vi "arm-sim-main.vi"() -> ()   [LabVIEW 2020]
uses:
  RobotCode/Arm/ArmPositionPreset.ctl
  RobotCode/Arm/ArmGamePiecePreset.ctl
  <vilib>/Rock Robotics/WPI/ThirdParty/JAS_Junk/TrajLib/Enum/DCMOTOR_TYPES_ENUM.ctl
  <vilib>/Analysis/Matrix/Datatypes/RealMatrix.ctl
  <vilib>/Rock Robotics/WPI/ThirdParty/JAS_Junk/TrajLib/DCMotor_GetCIM.vi
  <vilib>/Rock Robotics/WPI/ThirdParty/JAS_Junk/TrajLib/DCMotor_GetAndymark9015.vi
  <vilib>/Rock Robotics/WPI/ThirdParty/JAS_Junk/TrajLib/DCMotor_GetAndymarkRs775_125.vi
  <vilib>/Rock Robotics/WPI/ThirdParty/JAS_Junk/TrajLib/DCMotor_GetBag.vi
  <vilib>/Rock Robotics/WPI/ThirdParty/JAS_Junk/TrajLib/DCMotor_GetBanebotsRs550.vi
  <vilib>/Rock Robotics/WPI/ThirdParty/JAS_Junk/TrajLib/DCMotor_GetBanebotsRs775.vi
  <vilib>/Rock Robotics/WPI/ThirdParty/JAS_Junk/TrajLib/DCMotor_GetFalcon500.vi
  <vilib>/Rock Robotics/WPI/ThirdParty/JAS_Junk/TrajLib/DCMotor_GetMiniCIM.vi
  <vilib>/Rock Robotics/WPI/ThirdParty/JAS_Junk/TrajLib/DCMotor_GetNEO.vi
  <vilib>/Rock Robotics/WPI/ThirdParty/JAS_Junk/TrajLib/DCMotor_GetNEO550.vi
  <vilib>/Rock Robotics/WPI/ThirdParty/JAS_Junk/TrajLib/DCMotor_GetRomiBuiltIn.vi
  <vilib>/Rock Robotics/WPI/ThirdParty/JAS_Junk/TrajLib/DCMotor_GetVex775Pro.vi
  <vilib>/Rock Robotics/WPI/ThirdParty/JAS_Junk/TrajLib/VI/DCMotor_GetAndymarkAM2235A.vi
  <vilib>/Rock Robotics/WPI/ThirdParty/JAS_Junk/TrajLib/VI/DCMotor_GetAndymarkAM3493.vi
  <vilib>/Rock Robotics/WPI/ThirdParty/JAS_Junk/TrajLib/LinearFilter_ResetToValue.vi
  <vilib>/Rock Robotics/WPI/ThirdParty/JAS_Junk/TrajLib/LinearFilter_Calculate.vi
  <vilib>/Rock Robotics/WPI/ThirdParty/JAS_Junk/TrajLib/DCMotor_New.vi
  <vilib>/Rock Robotics/WPI/ThirdParty/JAS_Junk/TrajLib/VI/Units_RotationsPerMinuteToRadiansPerSecond.vi
  <vilib>/Analysis/Matrix/Numeric/Conversions/Array To Matrix - RA.vi
  arm-sim-subvi/arm-sim-globals.vi
  <vilib>/Rock Robotics/WPI/ThirdParty/JAS_Junk/TrajLib/LinearFilter_MovingAverage.vi
  <vilib>/Rock Robotics/WPI/ThirdParty/JAS_Junk/TrajLib/LinearFilter_LowPassBW1.vi
  <vilib>/Rock Robotics/WPI/ThirdParty/JAS_Junk/TrajLib/LinearFilter_LowPassBW2.vi
  <vilib>/Rock Robotics/WPI/ThirdParty/JAS_Junk/TrajLib/LinearFilter_HighPassBW1.vi
  <vilib>/Rock Robotics/WPI/ThirdParty/JAS_Junk/TrajLib/LinearFilter_HighPassBW2.vi
  <vilib>/Rock Robotics/WPI/ThirdParty/JAS_Junk/TrajLib/Trajectory_Library.lvlib
  <vilib>/Analysis/Matrix/NI_Matrix.lvlib
panel:
  in  "Execute Preset":bool
  in  "Game Piece":T1
  in  "Position":T2=enum."Middle"
  in  "Tab Control":T3(tab)
  out "Lift Control Chart":T4(graph)
  out "Extend Control Chart":T4(graph)
  out "Battery Volts, Current Chart":cluster{"Output":dbl, "Output":dbl}(graph)
  out "Lift Err":bool
  out "RLEOnTarget":bool
  out "Extend at Low\nLimit":bool
  out "Ext Pos Inches":dbl
  out "Ext Err":bool
  out "Total Amps":dbl format="%17.2f"
  out "battery voltge":dbl format="%14.2f"
  out "ArmAngle_Deg":dbl format="%20.1f"
  # "PRESET"
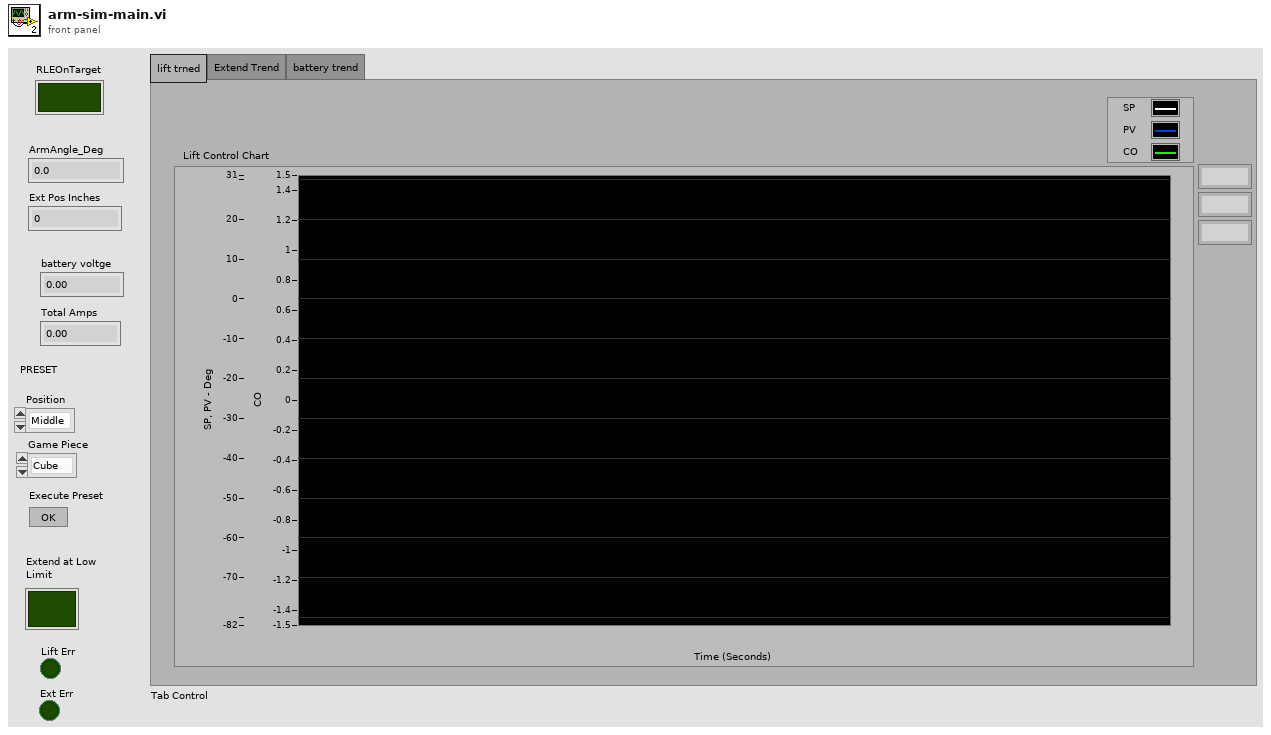
[diagram p1: front panel]
types:
  T1 = typedef "ArmGamePiecePreset.ctl" = enum16{"Cube", "Cone"}
  T2 = typedef "ArmPositionPreset.ctl" = enum16{"Upper", "Lower", "Middle", "Home", "Shelf", "Floor"}
  T3 = enum32{"lift trned", "Extend Trend", "battery trend"}
  T4 = cluster{"LiftPositionDemand(d)":dbl, "LiftPostion":dbl, "LiftMotorOutput":dbl}
  T5 = typedef "NI_Matrix.lvlib/RealMatrix.ctl" = dbl[][]
  T6 = typedef "Trajectory_Library.lvlib/DCMOTOR_TYPES_ENUM.ctl" = enum16{"CIM", "AndyMark 9015", "Andy Mark RS 775 125", "Bag", "BaneBots RS 550", "BaneBots RS 775", "Falcon 500", "Mini CIM", "NEO", "NEO 550", "Romi BuiltIn", "Vex 775 Pro", "Snow Blower AM 2235A", "Bosch Seat AM 3493"}
  T7 = typedef "Trajectory_Library.lvlib/DCMOTOR.CTL" = cluster{"nominalVoltage_Volts":dbl, "StallTorque_NM":dbl, "StallCurrent_Amps":dbl, "FreeCurrent_Amps":dbl, "FreeSpeed_RadPerSec":dbl, "R_Ohms":dbl, "KvINV_RadPerSecPerVolt":dbl, "Kt_NMPerAmp":dbl, "L_H":dbl, "Jr_KgM2":dbl}
  T8 = typedef "Trajectory_Library.lvlib/ELEVATOR_SIM.ctl" = cluster{"LinearSystemSim":T9, "GearBox":T7, "Gearing":dbl, "DrumRadius_M":dbl, "MinHeight_M":dbl, "MaxHeight_M":dbl, "CarriageMass_Kg":dbl, "SimulateGravity":bool}
  T9 = typedef "Trajectory_Library.lvlib/LINEAR_SYSTEM_SIM.ctl" = cluster{"m_Plant":T10, "m_X":T5, "m_Y":T5, "m_U":T5, "MeasureStdDev":T5}
  T10 = typedef "Trajectory_Library.lvlib/LINEAR_SYSTEM.ctl" = cluster{"m_A":T5, "m_B":T5, "m_C":T5, "m_D":T5, "States":i32, "Inputs":i32, "Outputs":i32}
  T11 = typedef "Trajectory_Library.lvlib/SINGLE_JOINT_ARM_SIM.ctl" = cluster{"Arm_LinearSystem":T9, "GearBox":T7, "Gearing":dbl, "R_ArmLength_M":dbl, "MinAngle_Rad":dbl, "MaxAngle_Rad":dbl, "SimulateGravity":bool}
  T12 = enum16{"Moving Average", "Low Pass 1st Order Butterworth", "Low Pass 2nd Order Butterworth", "High Pass 1st Order Butterworth", "High Pass 2nd Order Butterworth"}
  T13 = cluster{"ExtendPositonDemand(in)":dbl, "ExtendPostion":dbl, "ExtendMotorOutput":dbl}
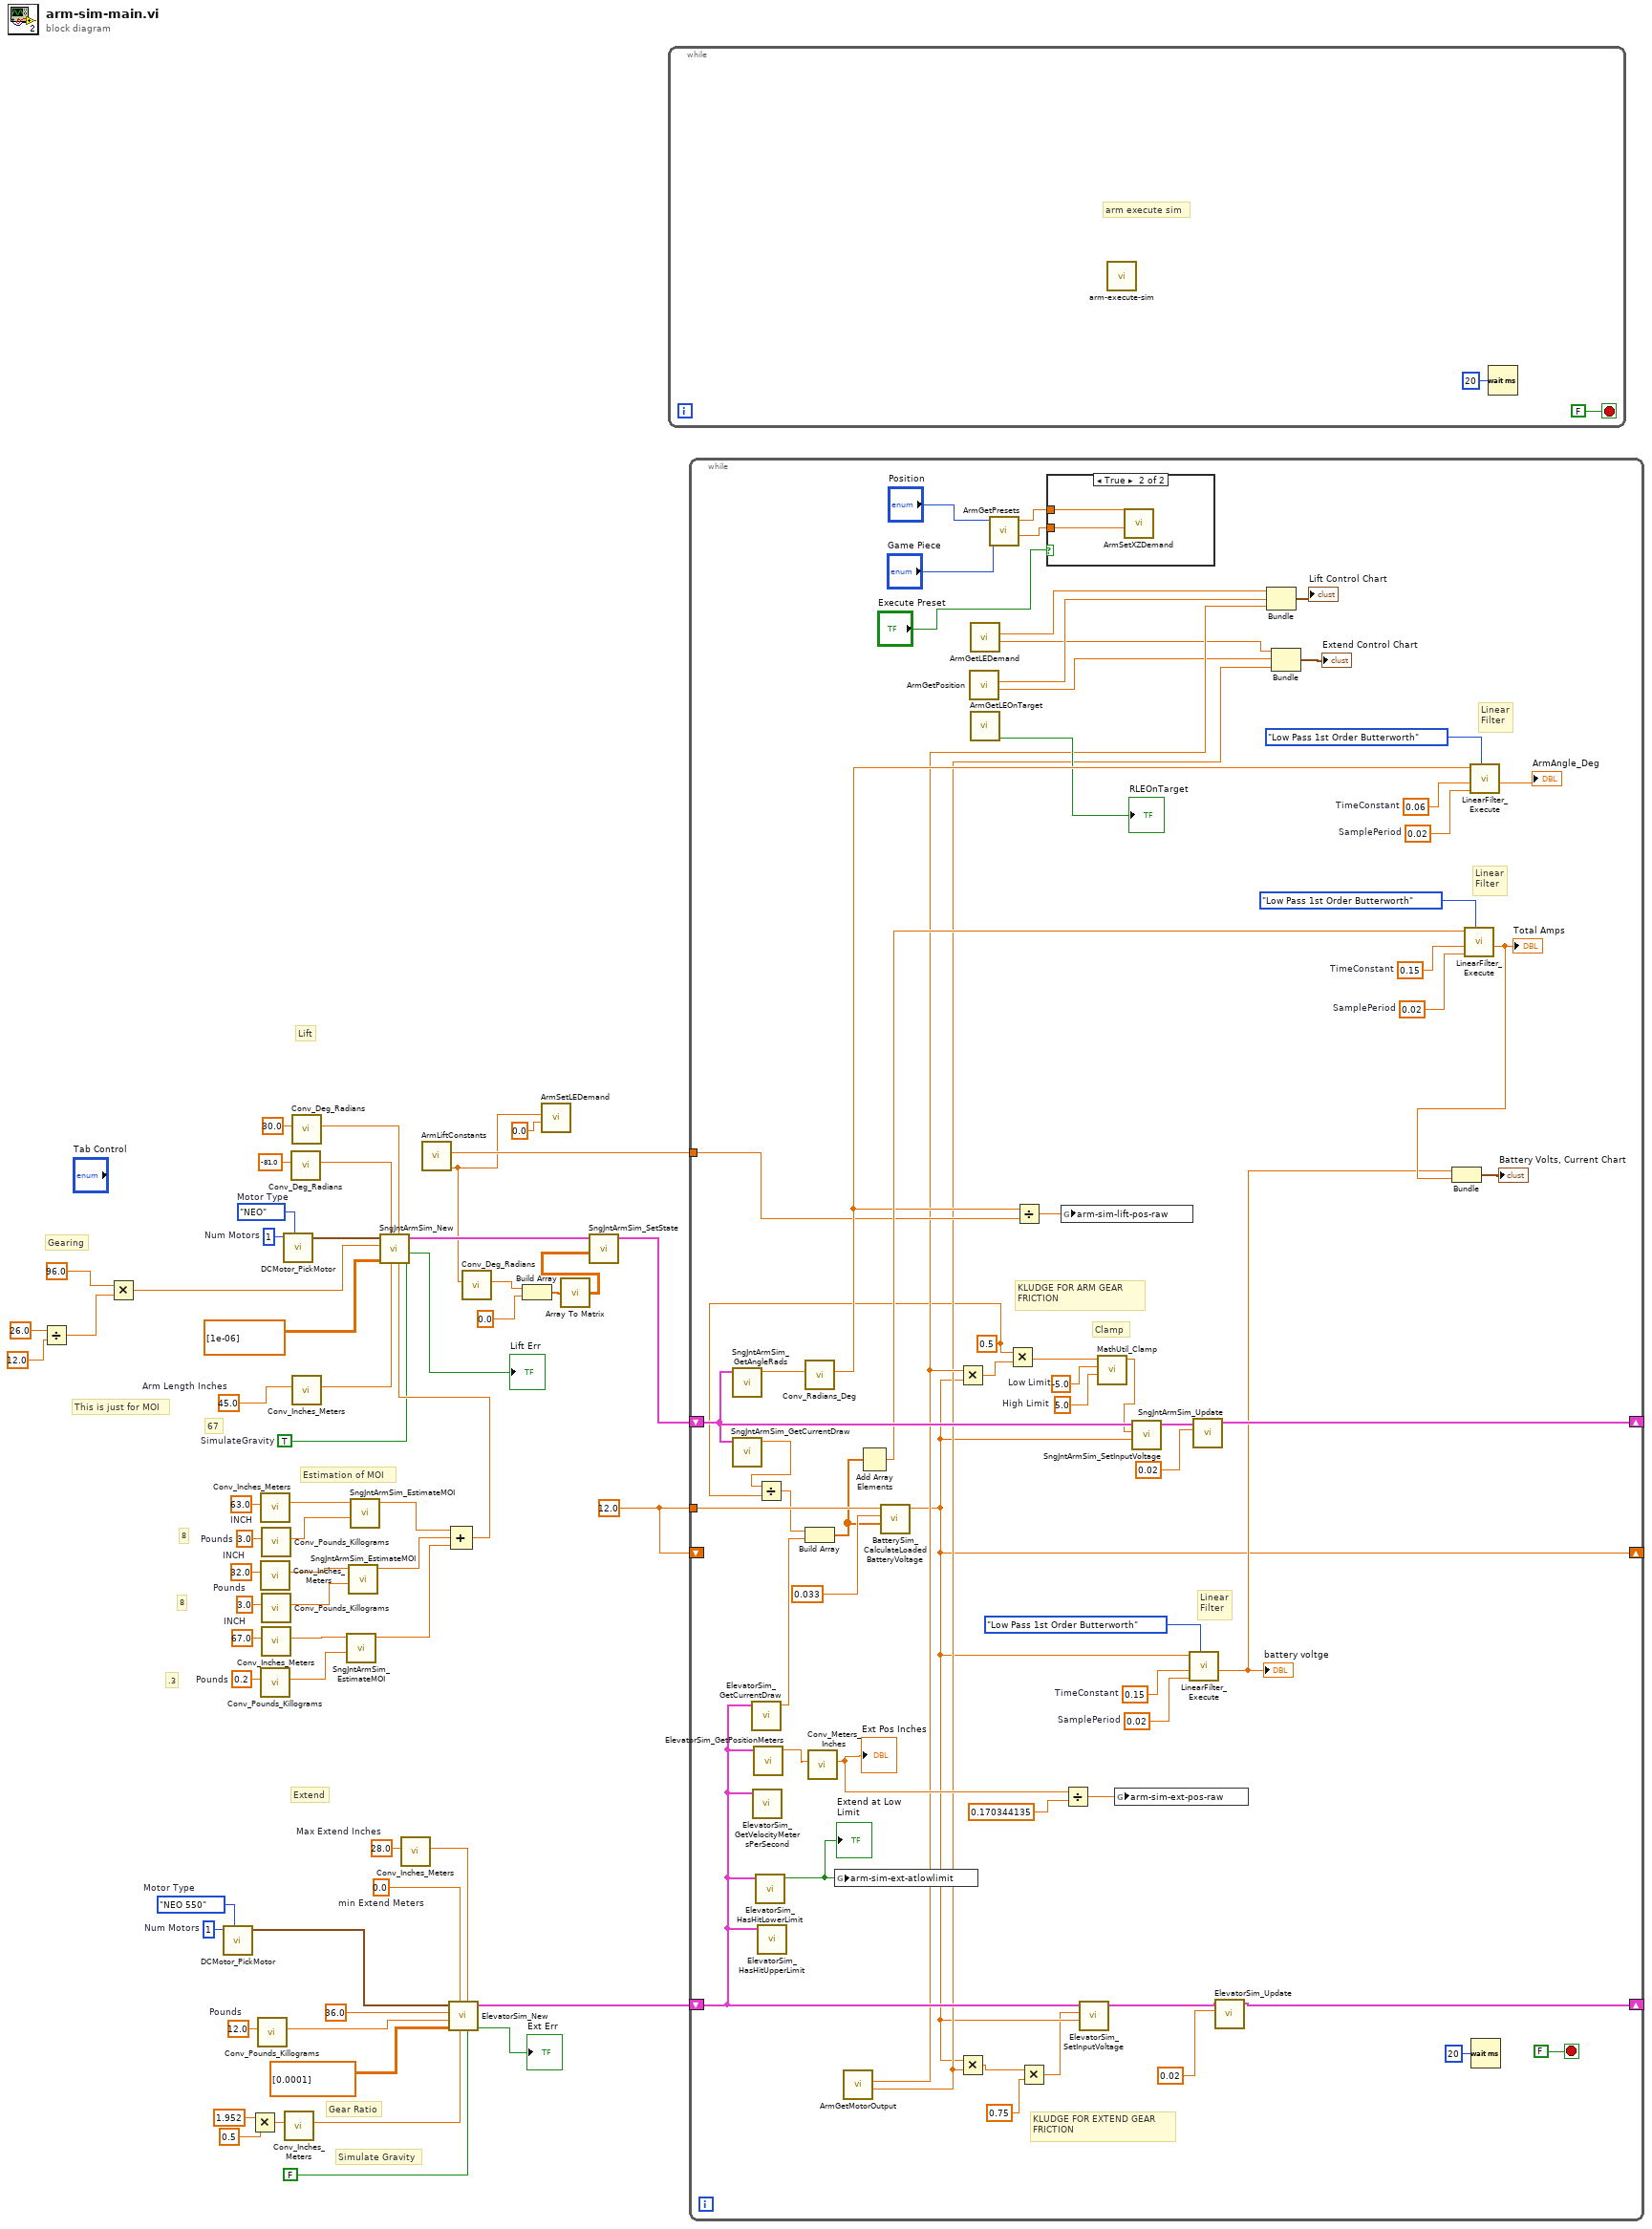
[diagram p0: block diagram]
diagram:
  w13 = 12.0  # Pounds
  w23 = 1  # Num Motors
  w22 = DCMOTOR_TYPES_ENUM."NEO 550"  # Motor Type
  w25 = 28.0  # Max Extend Inches
  w26 = 0.0  # min Extend Meters
  w35 = 12.0
  w40 = 3.0  # Pounds
  w41 = 3.0  # Pounds
  w42 = 0.2  # Pounds
  w43 = 67.0  # INCH
  w44 = 63.0  # INCH
  w45 = 32.0  # INCH
  w54 = TRUE  # SimulateGravity
  w57 = 45.0  # Arm Length Inches
  w60 = 1  # Num Motors
  w59 = DCMOTOR_TYPES_ENUM."NEO"  # Motor Type
  # "67"
  # "Simulate Gravity"
  # "Gear Ratio"
  # "Extend"
  # ".3"
  # "8"
  # "8"
  # "This is just for MOI"
  # "Estimation of MOI"
  # "Gearing"
  # "Lift"
  n1 = Divide(x=26.0, y=12.0) -> (x/y=w29:dbl)
  n2 = Multiply(x=96.0, y=w29) -> (x*y=w28:dbl)
  n3 = call <vilib>:"DCMotor_PickMotor.vi"("DCMOTOR_TYPES"=w22, "Num Motors"=w23) -> ("DCMOTOR"=w21:T7)  [unwired: 9 in]
  n4 = Multiply(x=1.952 ("INCH"), y=0.5) -> (x*y=w17:dbl)
  n5 = call <vilib>:"Conv_Pounds_Killograms.vi"("Pounds"=w13) -> ("Killograms"=w12:dbl)  [unwired: 10 in]
  n6 = call <vilib>:"Conv_Inches_Meters.vi"("INCH"=w44) -> ("Meters"=w53:dbl)  [unwired: 10 in]
  n7 = call <vilib>:"Conv_Inches_Meters.vi"("INCH"=w45) -> ("Meters"=w52:dbl)  [unwired: 10 in]
  n8 = call <vilib>:"Conv_Pounds_Killograms.vi"("Pounds"=w42) -> ("Killograms"=w50:dbl)  [unwired: 10 in]
  n9 = call <vilib>:"Conv_Pounds_Killograms.vi"("Pounds"=w40) -> ("Killograms"=w33:dbl)  [unwired: 10 in]
  n10 = call <vilib>:"Conv_Pounds_Killograms.vi"("Pounds"=w41) -> ("Killograms"=w49:dbl)  [unwired: 10 in]
  n11 = call <vilib>:"Conv_Inches_Meters.vi"("INCH"=w43) -> ("Meters"=w51:dbl)  [unwired: 10 in]
  n12 = call <vilib>:"DCMotor_PickMotor.vi"("DCMOTOR_TYPES"=w59, "Num Motors"=w60) -> ("DCMOTOR"=w58:T7)  [unwired: 9 in]
  n13 = call <vilib>:"Conv_Inches_Meters.vi"("INCH"=w17) -> ("Meters"=w16:dbl)  [unwired: 10 in]
  n14 = call <vilib>:"Conv_Deg_Radians.vi"("Degress"=-81.0) -> ("Radians"=w34:dbl)  [unwired: 10 in]
  n15 = call <vilib>:"Conv_Deg_Radians.vi"("Degress"=30.0) -> ("Radians"=w37:dbl)  [unwired: 10 in]
  n16 = call <vilib>:"Conv_Inches_Meters.vi"("INCH"=w57) -> ("Meters"=w56:dbl)  [unwired: 10 in]
  n17 = call <vilib>:"SngJntArmSim_EstimateMOI.vi"("ArmMass_Kg"=w50, "ArmLength_M"=w51) -> ("MOI"=w46:dbl)  [unwired: 9 in]
  n18 = call <vilib>:"SngJntArmSim_EstimateMOI.vi"("ArmMass_Kg"=w49, "ArmLength_M"=w52) -> ("MOI"=w47:dbl)  [unwired: 9 in]
  n19 = call <vilib>:"SngJntArmSim_EstimateMOI.vi"("ArmMass_Kg"=w33, "ArmLength_M"=w53) -> ("MOI"=w48:dbl)  [unwired: 9 in]
  n20 = call <vilib>:"Conv_Inches_Meters.vi"("INCH"=w25) -> ("Meters"=w24:dbl)  [unwired: 10 in]
  n21 = call "ArmLiftConstants.vi"() -> ("Starting Angle"=w2:dbl, "LiftConversionFactor"=w4:dbl)  [unwired: 8 in, 2 out]
  n22 = call <vilib>:"ElevatorSim_New.vi"("Simulate Gravity"=FALSE, "MaxHeight_Meters"=w24, "DrumRadius_Meters"=w16, "MinHeight_Meters"=w26, "MeasurementStdDev"=T5 [[0.0001]], "CarriageMass_Kg"=w12, "Gearing"=36.0, "GearBox"=w21) -> ("Error"=→"Ext Err":bool, "ElevatorSim"=w27:T8)  [unwired: 2 in]
  n23 = Compound Arithmetic op=ADD(w48, w47, w46) -> (w55:dbl)
  n24 = call <vilib>:"SngJntArmSim_New.vi"("SimulateGravity"=w54, "jKgMetersSquared"=w55, "MaxAngle_Rad"=w37, "ArmLength_Meters"=w56, "MinAngle_Rad"=w34, "MeasurementStdDev"=T5 [[1e-06]], "Gearing"=w28, "GearBox"=w58) -> ("Error"=→"Lift Err":bool, "SingleJointArmSim"=w10:T11)  [unwired: 2 in]
  n25 = call <vilib>:"Conv_Deg_Radians.vi"("Degress"=w2) -> ("Radians"=w8:dbl)  [unwired: 10 in]
  n26 = Build Array(w8, 0.0 ("element")) -> (w6:dbl[])
  n27 = call "ArmSetLEDemand.vi"("SetExtendPositonDemand(in)"=0.0, "SetLIftPostionDemand(d)"=w2) -> ()  [unwired: 10 in]
  n28 = call-poly <vilib>:"Array To Matrix.vi"("Real 1D Array"=w6) -> ("Real Matrix (Column Vector)"=w5:T5)
  n29 = call <vilib>:"SngJntArmSim_SetState.vi"("System State"=w5, "in ArmSim"=w10) -> ("out ArmSim"=w9:T11)  [unwired: 8 in, 1 out]
  n30 = while {
    stop <- FALSE stop-if-true
    # "arm execute sim"
    n31 = call "arm-execute-sim.vi"() -> ()  [unwired: 12 in]
    n32 = Wait (ms)(milliseconds to wait=u32 20) -> ()  [unwired: 1 out]
  }
  n33 = while {
    tunnel: w35 -> [w123]
    shift-right: [w74] -> _
    shift-left: w35 -> [_]
    shift-right: [w118] -> _
    shift-left: w9 -> [w121]
    shift-right: [w99] -> _
    shift-left: w27 -> [w102]
    tunnel: w4 -> [w92]
    stop <- FALSE stop-if-true
    w64 = 0.5 ("x")
    w70 = 5.0  # High Limit
    w69 = -5.0  # Low Limit
    w111 = 0.02  # SamplePeriod
    w110 = 0.15  # TimeConstant
    w114 = 0.02  # SamplePeriod
    w113 = 0.06  # TimeConstant
    w117 = 0.02  # SamplePeriod
    w116 = 0.15  # TimeConstant
    # "Clamp"
    # "KLUDGE FOR EXTEND GEAR \nFRICTION"
    # "KLUDGE FOR ARM GEAR \nFRICTION"
    # "Linear\nFilter"
    # "Linear\nFilter"
    # "Linear\nFilter"
    n34 = call <vilib>:"SngJntArmSim_GetAngleRads.vi"("SingleJointArmSim"=w121) -> ("ArmAngle_Rad"=w108:dbl)  [unwired: 10 in]
    n35 = call <vilib>:"SngJntArmSim_GetCurrentDraw.vi"("SingleJointArmSim"=w121) -> ("Current_Amps"=w65:dbl)  [unwired: 10 in]
    n36 = call <vilib>:"ElevatorSim_GetCurrentDraw.vi"("ElevatorSim"=w102) -> ("Current_Amps"=w103:dbl)  [unwired: 10 in]
    n37 = call <vilib>:"ElevatorSim_GetVelocityMetersPerSecond.vi"("ElevatorSim"=w102) -> ()  [unwired: 10 in, 1 out]
    n38 = call <vilib>:"ElevatorSim_GetPositionMeters.vi"("ElevatorSim"=w102) -> ("Position_Meters"=w97:dbl)  [unwired: 10 in]
    n39 = call <vilib>:"ElevatorSim_HasHitLowerLimit.vi"("ElevatorSim"=w102) -> ("AtLowLimit"=w98:bool)  [unwired: 10 in]
    "Extend at Low\nLimit" <- w98
    n40 = Divide(x=w65, y=w64) -> (x/y=w63:dbl)
    n41 = call <vilib>:"ElevatorSim_HasHitUpperLimit.vi"("ElevatorSim"=w102) -> ()  [unwired: 10 in, 1 out]
    n42 = call <vilib>:"Conv_Radians_Deg.vi"("Radians"=w108) -> ("Degrees"=w93:dbl)  [unwired: 10 in]
    n43 = Build Array(w63, w103) -> (w96:dbl[])
    n44 = call <vilib>:"Conv_Meters_Inches.vi"("Meters"=w97) -> ("Inches"=w90:dbl)  [unwired: 10 in]
    "Ext Pos Inches" <- w90
    n45 = global write "arm-sim-globals.vi" "arm-sim-ext-atlowlimit"(w98) -> ()
    n46 = call "ArmGetMotorOutput.vi"() -> ("ExtendMotorOutput"=w80:dbl, "LiftMotorOutput"=w84:dbl)  [unwired: 10 in]
    n47 = Add Array Elements(numeric array=w96) -> (sum=w95:dbl)
    n48 = call <vilib>:"BatterySim_CalculateLoadedBatteryVoltage.vi"("Currents"=w96, "Resistance_Ohms"=0.033, "NominalVoltage"=w123) -> ("Voltage"=w74:dbl)  [unwired: 8 in]
    n49 = Multiply(x=w84, y=w74) -> (x*y=w68:dbl)
    n50 = Multiply(x=w74, y=w80) -> (x*y=w73:dbl)
    n51 = call "ArmGetPosition.vi"() -> ("ExtendPostion"=w81:dbl, "LiftPostion"=w86:dbl)  [unwired: 10 in]
    n52 = call "ArmGetLEDemand.vi"() -> ("ExtendPositonDemand(in)"=w82:dbl, "LiftPositionDemand(d)"=w88:dbl)  [unwired: 10 in]
    n53 = call "ArmGetLEOnTarget.vi"() -> ("RLEOnTarget"=→"RLEOnTarget":bool)  [unwired: 11 in]
    n54 = call "ArmGetPresets.vi"("Game Piece"="Game Piece", "Position"="Position") -> ("z"=w75:dbl, "x"=w76:dbl)  [unwired: 8 in]
    n55 = Multiply(x=w64, y=w68) -> (x*y=w67:dbl)
    n56 = Divide(x=w93, y=w92) -> (x/y=w94:dbl)
    n57 = Multiply(x=w73, y=0.75 ("x")) -> (x*y=w71:dbl)
    n58 = case shown="True" "Execute Preset" {
      tunnel: w76 -> [_ w127]
      tunnel: w75 -> [_ w126]
      frame False {
      }
      frame True {
        n59 = call "ArmSetXZDemand.vi"("SetZ"=w126, "SetX"=w127) -> ()  [unwired: 10 in]
      }
    }
    n60 = global write "arm-sim-globals.vi" "arm-sim-lift-pos-raw"(w94) -> ()
    n61 = Divide(x=w90, y=0.170344135) -> (x/y=w91:dbl)
    n62 = call <vilib>:"ElevatorSim_SetInputVoltage.vi"("Battery_Volts"=w74, "Input_Voltage"=w71, "in ElevatorSim"=w102) -> ("out ElevatorSim"=w101:T8)  [unwired: 8 in]
    n63 = call <vilib>:"MathUtil_Clamp.vi"("High Limit"=w70, "Low Limit"=w69, "Value"=w67) -> ("Result"=w66:dbl)  [unwired: 8 in]
    n64 = global write "arm-sim-globals.vi" "arm-sim-ext-pos-raw"(w91) -> ()
    n65 = call <vilib>:"SngJntArmSim_SetInputVoltage.vi"("Battery_Volts"=w74, "Input_Voltage"=w66, "in SingleJointArmSim"=w121) -> ("out SingleJointArmSim"=w120:T11)  [unwired: 8 in]
    n66 = call <vilib>:"LinearFilter_Execute.vi"("Filter Type"=T12."Low Pass 1st Order Butterworth", "SamplePeriod"=w117, "TimeConstant"=w116, "Input"=w74) -> ("Output"=w104:dbl)  [unwired: 6 in, 1 out]
    "battery voltge" <- w104
    n67 = call <vilib>:"SngJntArmSim_Update.vi"("dT_Seconds"=0.02, "in SingleJointArmSim"=w120) -> ("out SingleJointArmSim"=w118:T11)  [unwired: 8 in, 1 out]
    n68 = call <vilib>:"ElevatorSim_Update.vi"("dT_Seconds"=0.02, "in ElevatorSim"=w101) -> ("out ElevatorSim"=w99:T8)  [unwired: 8 in, 1 out]
    n69 = Bundle("LiftPositionDemand(d)"=w88, "LiftPostion"=w86, "LiftMotorOutput"=w84) -> (→"Lift Control Chart":T4)  [unwired: 1 in]
    n70 = Bundle("ExtendPositonDemand(in)"=w82, "ExtendPostion"=w81, "ExtendMotorOutput"=w80) -> (→"Extend Control Chart":T13)  [unwired: 1 in]
    n71 = call <vilib>:"LinearFilter_Execute.vi"("Filter Type"=T12."Low Pass 1st Order Butterworth", "SamplePeriod"=w111, "TimeConstant"=w110, "Input"=w95) -> ("Output"=w105:dbl)  [unwired: 6 in, 1 out]
    "Total Amps" <- w105
    n72 = Bundle("Output"=w104, "Output"=w105) -> (→"Battery Volts, Current Chart":cluster{"Output":dbl, "Output":dbl})  [unwired: 1 in]
    n73 = call <vilib>:"LinearFilter_Execute.vi"("Filter Type"=T12."Low Pass 1st Order Butterworth", "SamplePeriod"=w114, "TimeConstant"=w113, "Input"=w93) -> ("Output"=→"ArmAngle_Deg":dbl)  [unwired: 6 in, 1 out]
    n74 = Wait (ms)(milliseconds to wait=u32 20) -> ()  [unwired: 1 out]
  }
